vi "chart series set labels separator.vi"(8 "error in (no error)":errorcluster, 10 "separator":u8, 11 "series":u32) -> (0 "error out":errorcluster)   [LabVIEW 2015, in "xlsxwriter.lvlib"]
doc: "void chart_series_set_labels_separator(lxw_chart_series series, uint8_t separator);"
uses:
  xlsxwriter.lvlib
  xlsxwriter.dll
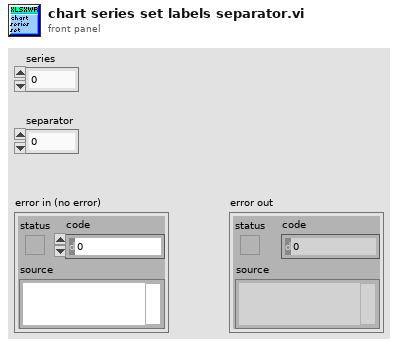
[diagram p1: front panel]
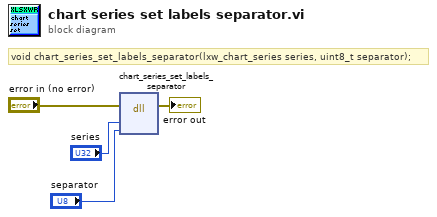
[diagram p0: block diagram]
diagram:
  # "void chart_series_set_labels_separator(lxw_chart_series series, uint8_t separator);"
  n1 = dll-call lib="C:/Users/WDAGUtilityAccount/Desktop/lv_vis_added_cell/xlsxwriter.*" fn="chart_series_set_labels_separator"(error in="error in (no error)", "series"="series", "separator"="separator") -> (error out=→"error out":errorcluster)  [unwired: 5 in, 1 out]
